vi "Experiment Diagram.vi"   [LabVIEW 2016]
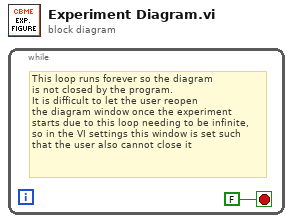
[diagram p0: block diagram]
diagram:
  n1 = while {
    stop <- FALSE stop-if-true
    # "This loop runs forever so the diagram \nis not closed by the program. \nIt is difficult to let the user reopen \nthe diagram window once the experiment \nstarts due to this loop needing to be infinite,\nso in the VI settings this window is set such \nthat the user also cannot close it"
  }
